vi "Edit GU Arrange.vi"(6 "Curr Cal Cfg In":T1, 8 "error in":errorcluster, 9 "Items Pre Edit":string[][](array[string]), 10 "Coords":T2, 11 "CtlRef":refnum<vi>) -> (0 "error out":errorcluster)   [LabVIEW 2020, in "GUCalibration2.lvlib"]
uses:
  GUCalibration2.lvlib
  <vilib>/Utility/miscctls.llb/LVRowAndColumnTypeDef.ctl
  Controls/Config Data Type.ctl
  Controls/User Facing Msg Enum.ctl
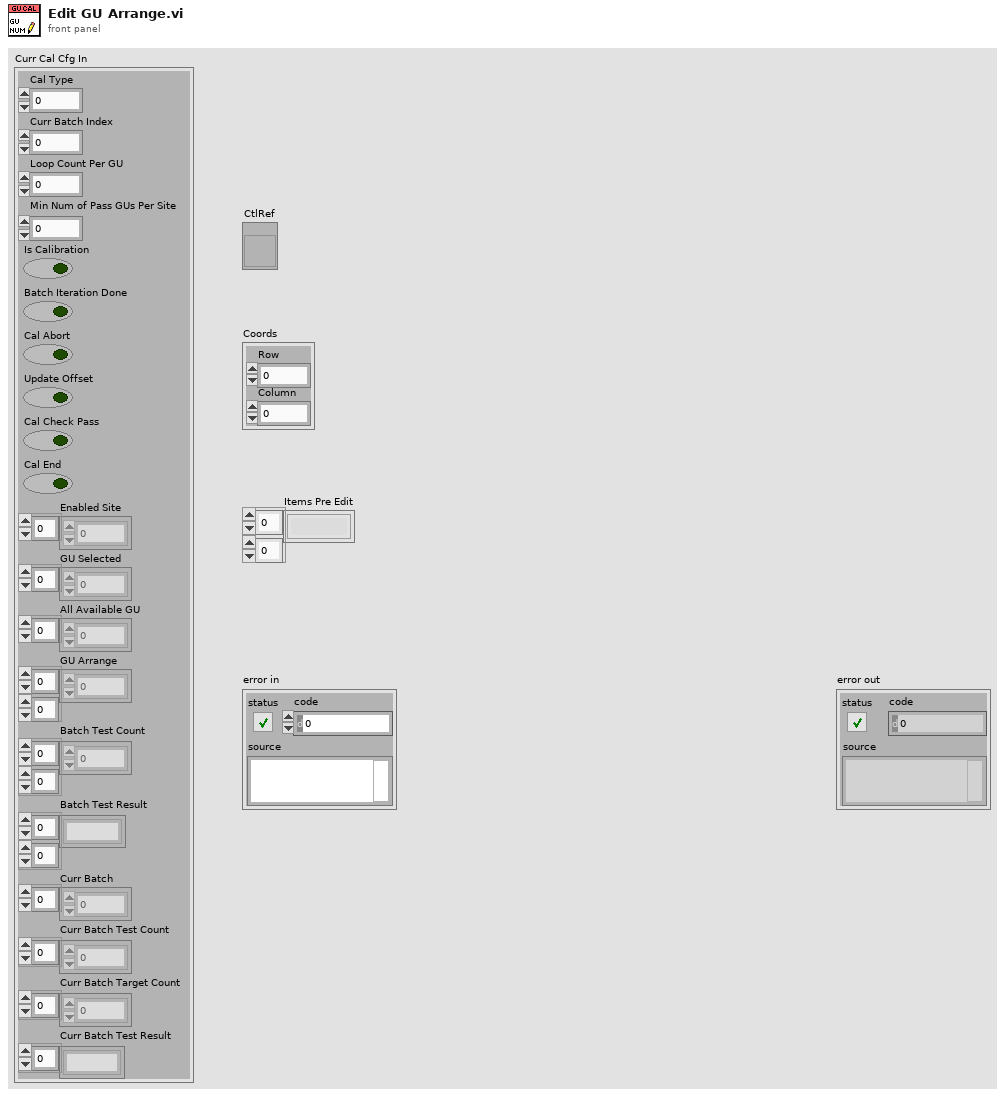
[diagram p1: front panel]
types:
  T1 = typedef "GUCalibration2.lvlib/Config Data Type.ctl" = cluster{"Cal Type":i32, "Curr Batch Index":i32, "Loop Count Per GU":i32, "Min Num of Pass GUs Per Site":i32, "Is Calibration":bool, "Batch Iteration Done":bool, "Cal Abort":bool, "Update Offset":bool, "Cal Check Pass":bool, "Cal End":bool, "Enabled Site":i32[], "GU Selected":i32[], "All Available GU":i32[], "GU Arrange":i32[][], "Batch Test Count":i32[][], "Batch Test Result":string[][], "Curr Batch":i32[], "Curr Batch Test Count":i32[], "Curr Batch Target Count":i32[], "Curr Batch Test Result":string[]}
  T2 = typedef "LVRowAndColumnTypeDef.ctl" = cluster{"Row":i32, "Column":i32}
  T3 = typedef "GUCalibration2.lvlib/User Facing Msg Enum.ctl" = enum16{"Invalid GU Number", "Select More GU", "Exceptional Lot End", "Not All Sites Test", "GU Arrange Error", "Put GU In Sites", "No Cal Site Offset Msg"}
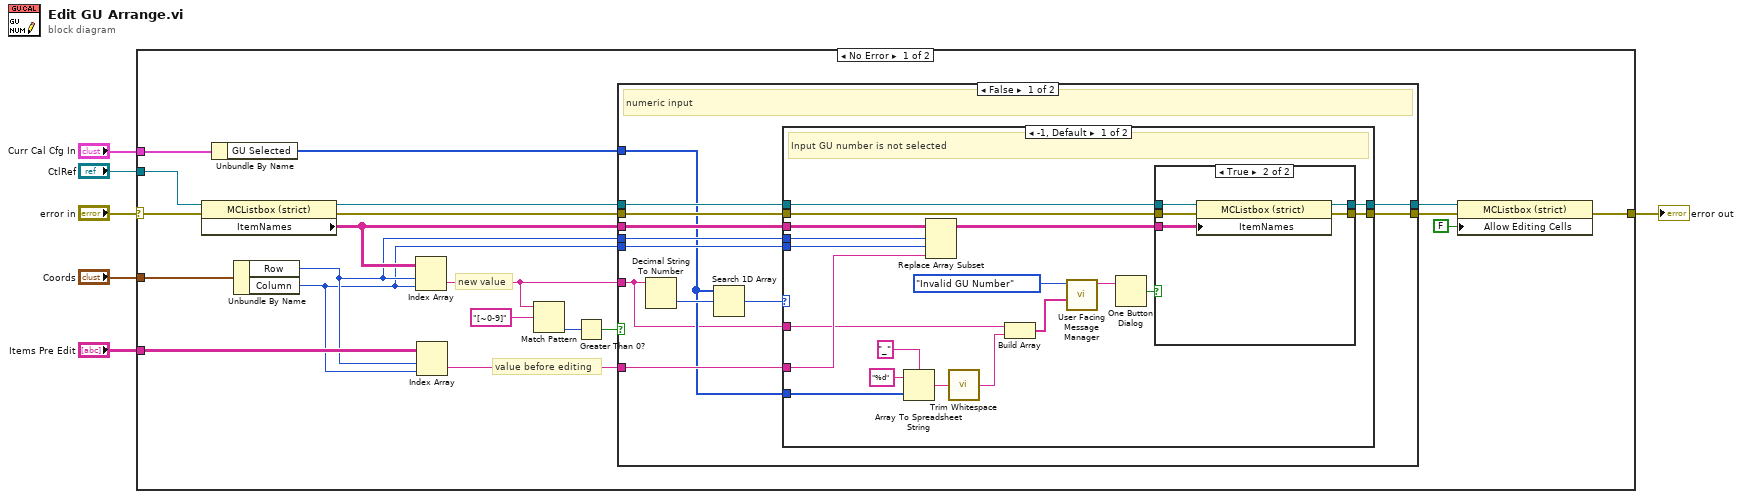
[diagram p0: block diagram]
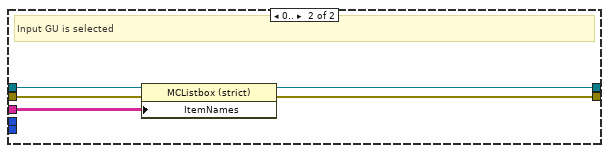
[diagram p3: hidden frame]
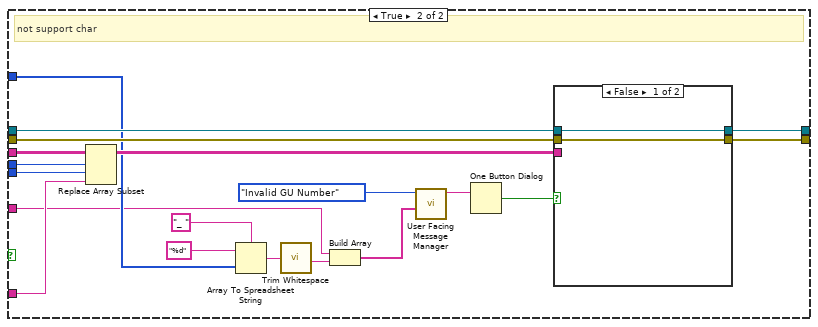
[diagram p4: hidden frame]
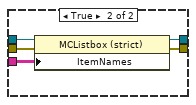
[diagram p5: hidden frame]
diagram:
  n1 = case shown="No Error" "error in" {
    selector: "error in" -> [w12 w96]
    tunnel: "CtlRef" -> [w25 _]
    tunnel: "Coords" -> [w11 _]
    tunnel: "Items Pre Edit" -> [w26 _]
    tunnel: "Curr Cal Cfg In" -> [w24 _]
    tunnel: [w8 w96] -> w2
    frame No Error {
      # "new value"
      # "value before editing"
      n2 = property class="MCListbox (strict)"(reference=w25, error in=w12) -> (reference out=w18:refnum<vi>, error out=w19:errorcluster, "ItemNames"=w20:string[][])
      n3 = Unbundle By Name(w24) -> ("GU Selected"=w14:i32[])
      n4 = Unbundle By Name(w11) -> ("Row"=w16:i32, "Column"=w15:i32)
      n5 = Index Array(array=w20, index (row)=w16, index (col)=w15) -> (element=w13:string)
      n6 = Index Array(array=w26, index (row)=w16, index (col)=w15) -> (element=w17:string)
      n7 = Match Pattern(string=w13, regular expression="[~0-9]") -> (offset past match=w22:i32)  [unwired: 1 in, 3 out]
      n8 = Greater Than 0?(x=w22) -> (x > 0?=w21:bool)
      n9 = case shown="False" w21 {
        tunnel: w20 -> [w34 w86]
        tunnel: w19 -> [w38 w88]
        tunnel: w18 -> [w36 w87]
        tunnel: w17 -> [w31 w85]
        tunnel: w16 -> [w33 w84]
        tunnel: w15 -> [w32 w83]
        tunnel: [w35 w81] -> w10
        tunnel: w14 -> [w29 w77]
        tunnel: w13 -> [w28 w72]
        tunnel: [w27 w75] -> w9
        frame False {
          # "numeric input"
          n10 = Decimal String To Number(string=w28) -> (number=w30:i32)  [unwired: 2 in, 1 out]
          n11 = Search 1D Array(1D array=w29, element=w30) -> (index of element=w37:i32)  [unwired: 1 in]
          n12 = case shown="-1, Default" w37 {
            tunnel: w38 -> [w57 w69]
            tunnel: w36 -> [w56 w68]
            tunnel: [w55 w67] -> w35
            tunnel: w34 -> [w54 w66]
            tunnel: w33 -> [w52 _]
            tunnel: w32 -> [w51 _]
            tunnel: w31 -> [w53 _]
            tunnel: w29 -> [w49 _]
            tunnel: w28 -> [w43 _]
            tunnel: [w44 w65] -> w27
            frame -1, Default {
              # "Input GU number is not selected"
              n13 = Array To Spreadsheet String(delimiter (Tab)="_", array=w49, 3:"%d" ("format string")) -> (spreadsheet string=w46:string)
              n14 = Replace Array Subset(array=w54, new element=w53, index (row)=w52, index (col)=w51) -> (w50:string[][])
              n15 = call <vilib>:"Trim Whitespace.vi"("string"=w46) -> ("trimmed string"=w42:string)  [unwired: 1 in]
              n16 = Build Array(w43, w42) -> (w41:string[])
              n17 = call "User Facing Message Manager.vi"("Variable Msg"=w41, "User Facing Msg"=User_Facing_Msg_Enum."Invalid GU Number") -> ("User Facing Msg Out"=w39:string)  [unwired: 7 in, 2 out]
              n18 = One Button Dialog(message=w39) -> (true=w45:bool)  [unwired: 1 in]
              n19 = case shown="True" w45 {
                tunnel: w57 -> [w59 w64]
                tunnel: w56 -> [w58 w63]
                tunnel: [w59 w62] -> w55
                tunnel: w50 -> [_ w61]
                tunnel: [w58 w60] -> w44
                frame False {
                }
                frame True {
                  n20 = property class="MCListbox (strict)"(reference=w63, error in=w64, "ItemNames"=w61) -> (reference out=w60:refnum<vi>, error out=w62:errorcluster)
                }
              }
            }
            frame 0.. {
              # "Input GU is selected"
              n21 = property class="MCListbox (strict)"(reference=w68, error in=w69, "ItemNames"=w66) -> (reference out=w65:refnum<vi>, error out=w67:errorcluster)
            }
          }
        }
        frame True {
          # "not support char"
          n22 = Replace Array Subset(array=w86, new element=w85, index (row)=w84, index (col)=w83) -> (w82:string[][])
          n23 = Array To Spreadsheet String(delimiter (Tab)="_ ", array=w77, 3:"%d" ("format string")) -> (spreadsheet string=w78:string)
          n24 = call <vilib>:"Trim Whitespace.vi"("string"=w78) -> ("trimmed string"=w71:string)  [unwired: 1 in]
          n25 = Build Array(w72, w71) -> (w74:string[])
          n26 = call "User Facing Message Manager.vi"("Variable Msg"=w74, "User Facing Msg"=User_Facing_Msg_Enum."Invalid GU Number") -> ("User Facing Msg Out"=w70:string)  [unwired: 7 in, 2 out]
          n27 = One Button Dialog(message=w70) -> (true=w76:bool)  [unwired: 1 in]
          n28 = case shown="False" w76 {
            tunnel: w88 -> [w90 w95]
            tunnel: w87 -> [w89 w94]
            tunnel: w82 -> [_ w93]
            tunnel: [w90 w92] -> w81
            tunnel: [w89 w91] -> w75
            frame False {
            }
            frame True {
              n29 = property class="MCListbox (strict)"(reference=w94, error in=w95, "ItemNames"=w93) -> (reference out=w91:refnum<vi>, error out=w92:errorcluster)
            }
          }
        }
      }
      n30 = property class="MCListbox (strict)"(reference=w9, error in=w10, "Allow Editing Cells"=FALSE) -> (error out=w8:errorcluster)  [unwired: 1 out]
    }
    frame Error {
    }
  }
  "error out" <- w2
